vi "计算三角形外心与半径.vi"(11 "三角形":T1) -> (2 "半径":dbl, 3 "外心":T2)   [LabVIEW 2012, in "几何工具.lvlib"]
uses:
  <vilib>/Utility/miscctls.llb/LVPointDoubleTypeDef.ctl
panel:
  out "Error Out":errorcluster caption="错误输出"
  in  "Error In":errorcluster caption="错误输入"
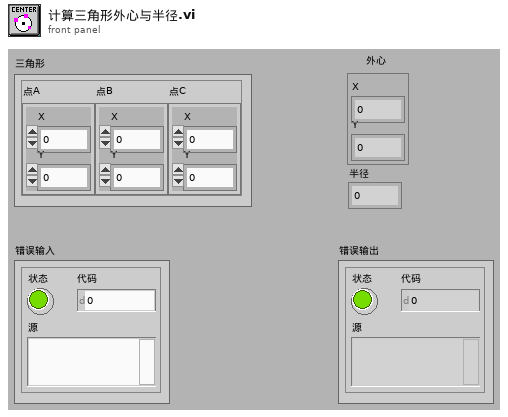
[diagram p1: front panel]
types:
  T1 = typedef "几何工具.lvlib/三角形.ctl" = cluster{"点A":T2, "点B":T2, "点C":T2}
  T2 = typedef "LVPointDoubleTypeDef.ctl" = cluster{"X":dbl, "Y":dbl}
  T3 = typedef "几何工具.lvlib/斜率与截距.ctl" = cluster{"斜率":dbl, "截距":dbl}
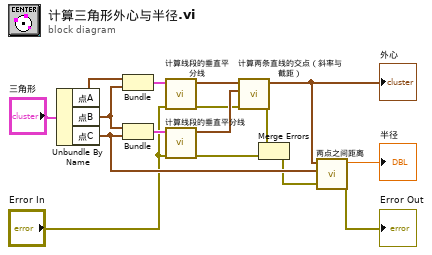
[diagram p0: block diagram]
diagram:
  n1 = Unbundle By Name("三角形") -> ("点A"=w7:T2, "点B"=w13:T2, "点C"=w9:T2)
  n2 = Bundle("点A"=w7, "点B"=w13) -> (w14:cluster{"点A":T2, "点B":T2})  [unwired: 1 in]
  n3 = Bundle("点B"=w13, "点C"=w9) -> (w12:cluster{"点B":T2, "点C":T2})  [unwired: 1 in]
  n4 = call "计算线段的垂直平分线.vi"("Error In"="Error In", "线段"=w14) -> ("Error Out"=w5:errorcluster, "斜率与截距"=w11:T3)  [unwired: 8 in]
  n5 = call "计算线段的垂直平分线.vi"("Error In"="Error In", "线段"=w12) -> ("Error Out"=w3:errorcluster, "斜率与截距"=w10:T3)  [unwired: 8 in]
  n6 = call "计算两条直线的交点（斜率与截距）.vi"("Error In"=w5, "直线B"=w10, "直线A"=w11) -> ("Error Out"=w4:errorcluster, "交点"=w8:T2)  [unwired: 7 in]
  "外心" <- w8
  n7 = Merge Errors(w4, w3) -> (w2:errorcluster)
  n8 = call "两点之间距离.vi"("Error In"=w2, "点B"=w9, "点A"=w8) -> ("Error Out"=→"Error Out":errorcluster, "距离AB"=→"半径":dbl)  [unwired: 7 in]
